vi "Example_OE2052 Control.vi"() -> ()   [LabVIEW 2011]
uses:
  <vilib>/Utility/error.llb/DialogType.ctl
panel:
  out "B_Freq":dbl
  out "B_θ":dbl
  out "B_R":dbl
  out "B_Overload":bool
  in  "Sample count":u32
  out "Zero Data?":bool
  in  "buffer":u8
  out "Queue out":errorcluster caption="error out"
  out "Queue output":refnum<queue>
  in  "IP Address":string
  in  "Timeout":u32=100
  in  "Port":u32=10001
  out "B_PLL Lock":bool
  in  "Remote Mode":u16(ring) items=["USB"=0, "RS232"=1, "Ethernet"=3]
  out "A_Freq":dbl
  out "A_θ":dbl
  out "A_R":dbl
  out "A_PLL Lock":bool
  out "A_Overload":bool
  out "Error":string
  out "Serial Versions":string
  in  "Table":T1(tab) caption="选项卡控件"
  in  "OE2052_Configure Input Filter":T2={"Input Source"=0, "Input Impedance"=0, "Input Coupling "=0, "Sample Mode"=0, "Channel"=1, "Input Range"=0} {"Input Range" items=["1.3V", "200mV", "50mV", "10mV", "2mV", "500uV", "100uV"]; "Channel" items=["A"=1, "B"=2]; "Sample Mode" items=["HF", "LF"]; "Input Coupling" items=["AC", "DC"]; "Input Impedance" items=["50Ω", "10MΩ"]; "Input Source" items=["A", "A-B"]}
  in  "OE2052_Configure Ref Phase":T3={"Reference Source"=0, "Internal Frequency(Hz)"=1000.0, "Reference Phase"=0.0, "Reference Slope"=0, "Channel"=1, "Reference Range"=0} {"Reference Range" items=["HIGH", "LOW"]; "Channel" items=["A"=1, "B"=2]; "Reference Slope" items=["SINEDC", "SINE", "TTL"]; "Reference Phase" min=-180.0 max=180.0 format="%#.2g"; "Internal Frequency(Hz)" min=1e-05 max=60000000.0 format="%#.3f"; "Reference Source" items=["External", "Internal", "Self"]}
  in  "OE2052_Configure \nGain TC":T4={"Time Constant "=20.0, "Low Pass Filter Slope "=3, "Enable Sync Filter "=0, "Channel"=1} {"Channel" items=["A"=1, "B"=2]; "Enable Sync Filter" items=["OFF", "ON"]; "Low Pass Filter Slope" items=["6 dB/oct", "12 dB/oct", "18 db/oct", "24 dB/oct", "30 dB/oct", "36 dB/oct", "42 dB/oct", "48 dB/oct"]; "Time Constant" min=1e-07 max=100.0 format="%#.3f"}
  in  "OE2052_Configure Channel Out":T5={"Channel Output"=0, "Channel Source"=0, "Offset(%)"=0.0, "Expand"=1, "AUX OUT"=1.0, "Sensitivity "=24} {"Sensitivity" items=["1 nV/fA", "2 nV/fA", "5 nV/fA", "10 nV/fA", "20 nV/fA", "50 nV/fA", "100 nV/fA", "200 nV/fA", "500 nV/fA", "1 uV/pA", "2 uV/pA", "5 uV/pA", "10 uV/pA", "20 uV/pA", "50 uV/pA", "100 uV/pA", "200 uV/pA", "500 uV/pA", "1 mV/nA", "2 mV/nA", "5 mV/nA", "10 mV/nA", "20 mV/nA", "50 mV/nA", "100 mV/nA", "200 mV/nA", "500 mV/nA", "1 V/uA"]; "AUX OUT" min=-10.0 max=10.0 format="%#.3g"; "Expand" min=1 max=10000; "Offset(%)" min=-100.0 max=100.0 format="%#_5g"; "Channel Source" items=["AUXOUT", "X1", "Y1", "R1", "θ1", "X2", "Y2", "R2", "θ2", "Frequency1", "Frequency2", "AUX-IN1", "AUX-IN2", "AUX-IN3", "AUX-IN4"]; "Channel Output" items=["CH1", "CH2", "CH3", "CH4"]}
  in  "OE2052_Configure Sine Out":T6={"SineOut Amplitude (V)"=1.0, "SineOut Offset(V) "=1.0, "SineOut Unit"=0, "SineOut Impedance"=0, "Channel"=1, "SineOut Mode"=0} {"SineOut Mode" items=["OFF", "Fixed"]; "Channel" items=["A"=1, "B"=2]; "SineOut Impedance" items=["50Ω", "HiZ"]; "SineOut Unit" items=["VPP", "VRMS"]; "SineOut Offset(V)" min=-2.5 max=2.5 format="%#.3g"; "SineOut Amplitude (V)" min=1e-06 max=1.5 format="%#.3g"}
  in  "OE2052_Configure Demodulator":T7={"Mode"=0, "Harmonic"=1, "Channel"=1} {"Channel" items=["A"=1, "B"=2]; "Harmonic" min=1; "Mode" items=["Harmonic"]}
  in  "OE2052_Auto Setting":T8={"Auto Range"=FALSE, "Auto Offest"=FALSE, "Auto Phase"=FALSE, "channel"=1} {"channel" items=["A"=1, "B"=2]}
  in  "Save Button":bool
  in  "file path":path
  in  "Sample Rate(S)":dbl=0.1 min=0.001 max=100.0
  out "Status":string
  in  "Connect":bool
  in  "VISA resource name":refnum<visa-resource-name>
  in  "Baud Rate (115200)":u32=921600
  # "Tel          :   +86-020-84133345\nWebsite  :   www.ssi-instrument.com\nE-mail     :   support@si-instrument.com"
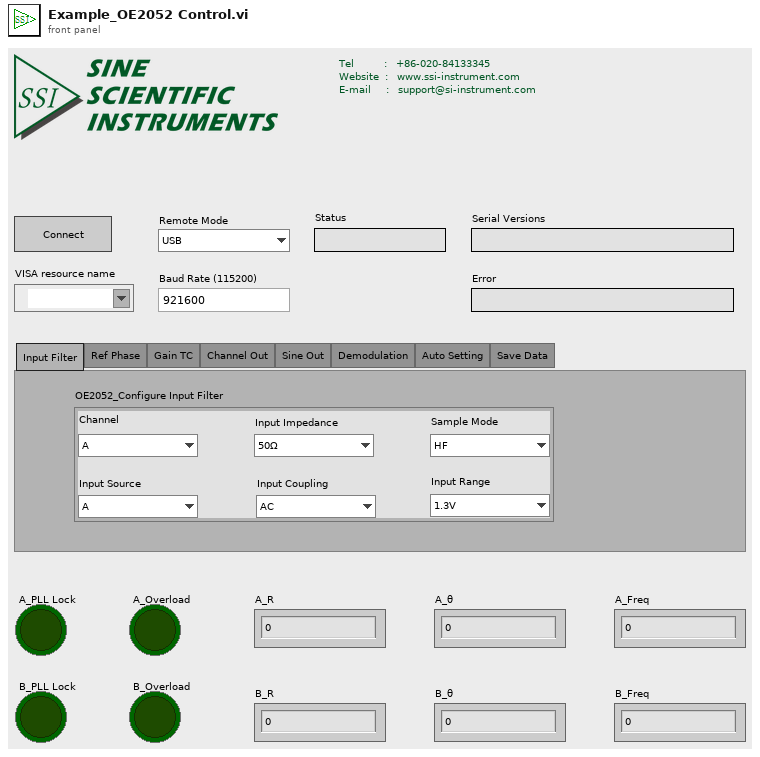
[diagram p1: front panel]
types:
  T1 = enum32{"Input Filter", "Ref Phase", "Gain TC", "Channel Out", "Sine Out", "Demodulation", "Auto Setting", "Save Data"}
  T2 = cluster{"Input Source":u16, "Input Impedance":u16, "Input Coupling ":u16, "Sample Mode":u16, "Channel":u16, "Input Range":u16}
  T3 = cluster{"Reference Source":u16, "Internal Frequency(Hz)":dbl, "Reference Phase":dbl, "Reference Slope":u16, "Channel":u16, "Reference Range":u16}
  T4 = cluster{"Time Constant ":dbl, "Low Pass Filter Slope ":u8, "Enable Sync Filter ":u16, "Channel":u16}
  T5 = cluster{"Channel Output":u16, "Channel Source":u16, "Offset(%)":dbl, "Expand":u16, "AUX OUT":dbl, "Sensitivity ":u16}
  T6 = cluster{"SineOut Amplitude (V)":dbl, "SineOut Offset(V) ":dbl, "SineOut Unit":u8, "SineOut Impedance":u8, "Channel":u16, "SineOut Mode":u8}
  T7 = cluster{"Mode":u16, "Harmonic":u16, "Channel":u16}
  T8 = cluster{"Auto Range":bool, "Auto Offest":bool, "Auto Phase":bool, "channel":u16}
  T9 = enum16{"OE1022", "OE1022D", "OE1201", "OE2031&OE2041", "OE1311&OE1351", "OE2052"}
  T10 = cluster{"Port":u32, "Timeout":u32, "IP Address":string}
  T11 = cluster{"A_PLL Lock":bool, "A_Overload":bool, "B_PLL Lock":bool, "B_Overload":bool}
  T12 = cluster{"A_X":dbl, "A_Y":dbl, "A_R":dbl, "A_θ":dbl, "A_Freq":dbl, "B_X":dbl, "B_Y":dbl, "B_R":dbl, "B_θ":dbl, "B_Freq":dbl, "Aux_In1":dbl, "Aux_In2":dbl, "Aux_In3":dbl, "Aux_In4":dbl}
  T13 = typedef "DialogType.ctl" = u16
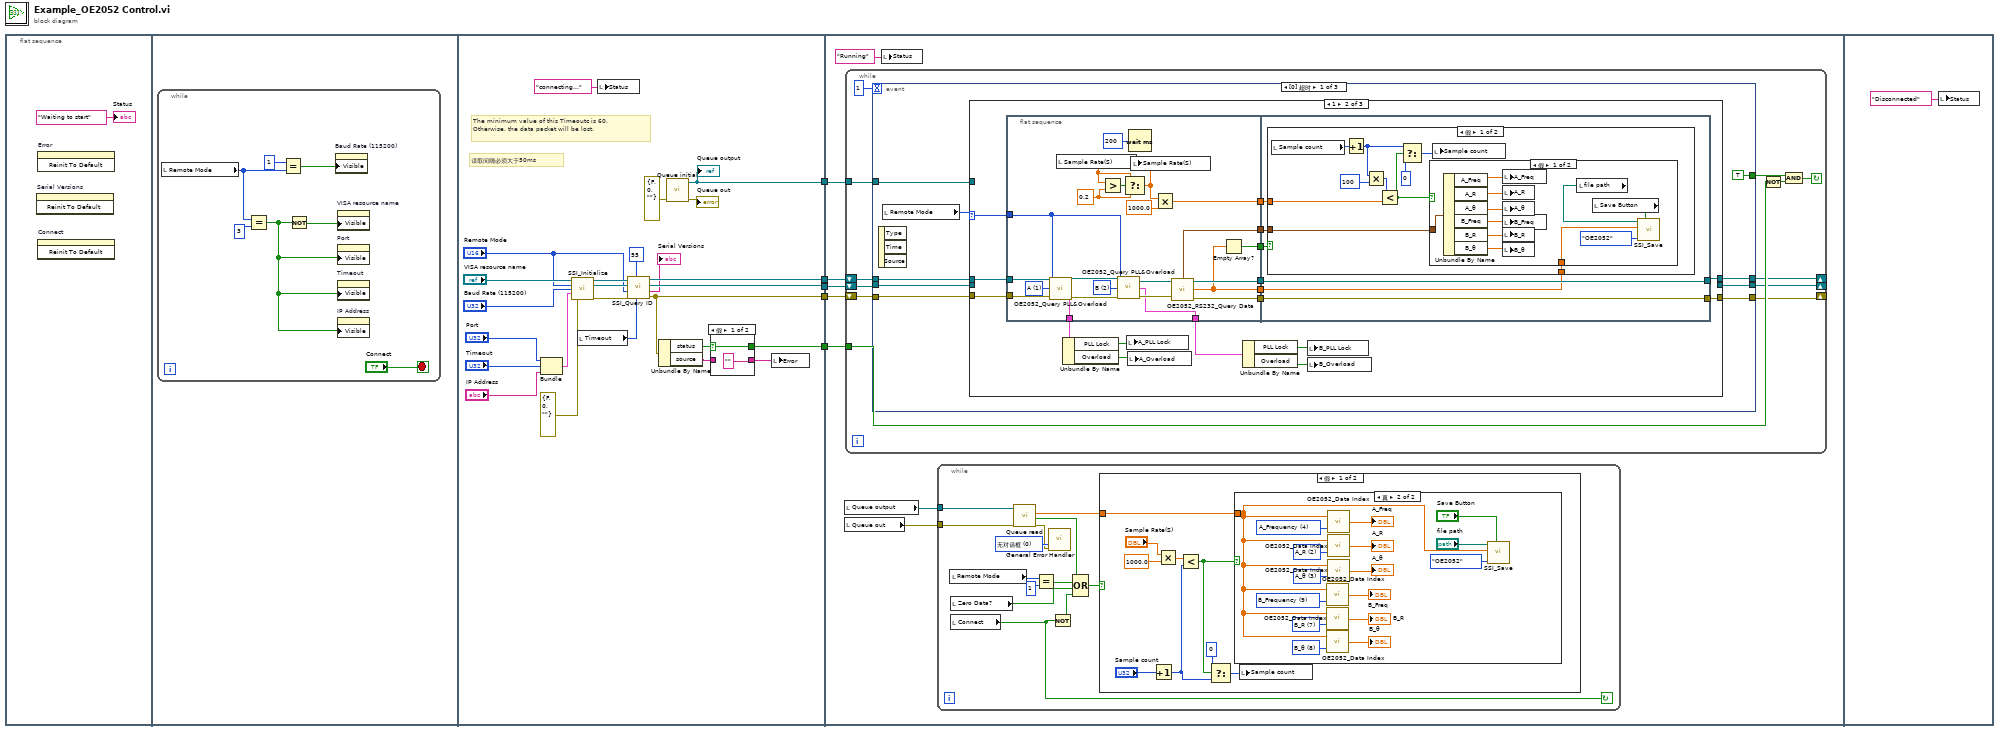
[diagram p0: block diagram]
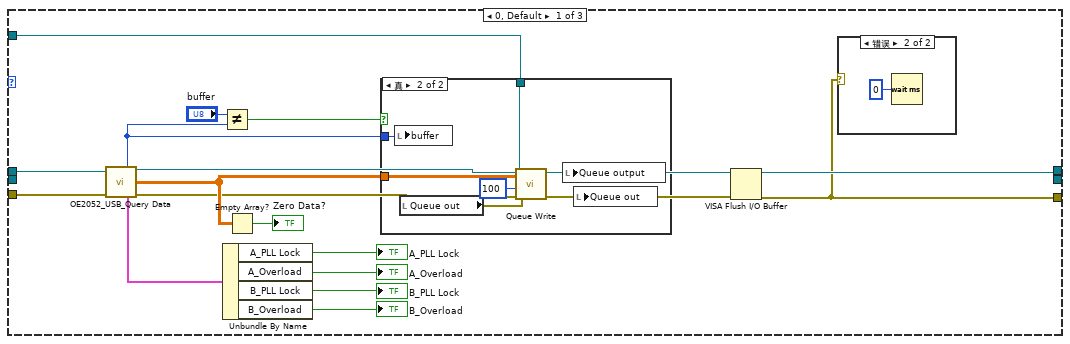
[diagram p5: hidden frame]
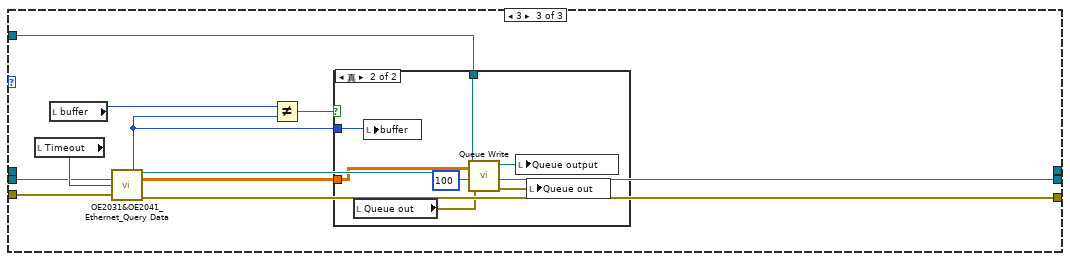
[diagram p10: hidden frame]
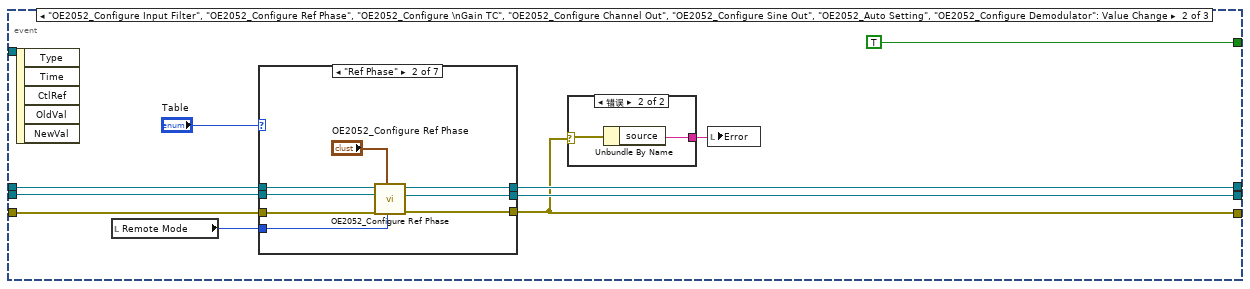
[diagram p12: hidden frame]
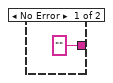
[diagram p13: hidden frame]
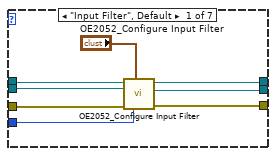
[diagram p14: hidden frame]
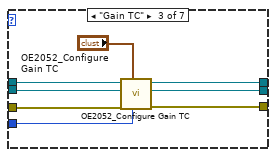
[diagram p15: hidden frame]
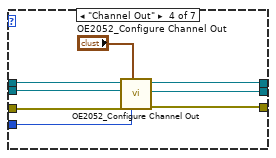
[diagram p16: hidden frame]
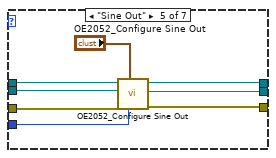
[diagram p17: hidden frame]
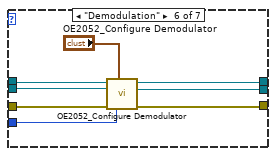
[diagram p18: hidden frame]
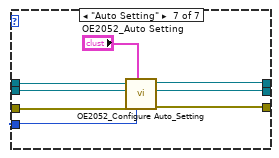
[diagram p19: hidden frame]
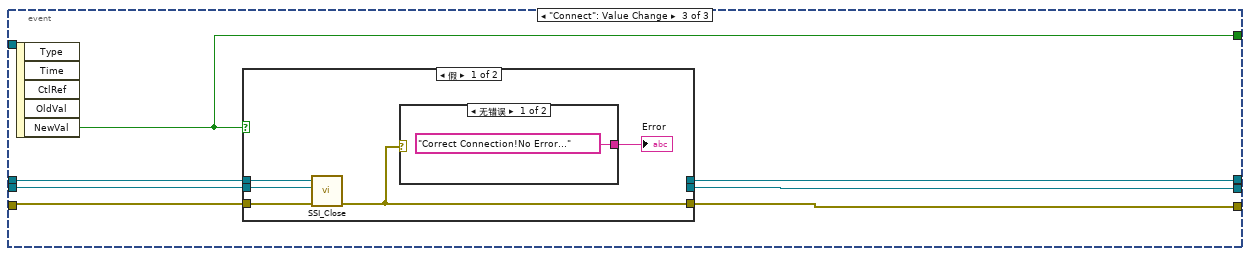
[diagram p20: hidden frame]
diagram:
  n1 = flat-sequence {
    tunnel: [w32] -> w5
    tunnel: [w31] -> w4
    tunnel: [w28] -> w3
    tunnel: [w25] -> w2
    tunnel: [w16] -> w1
    tunnel: w5 -> [w49]
    tunnel: w4 -> [w48]
    tunnel: w3 -> [w47]
    tunnel: w2 -> [w46]
    tunnel: w1 -> [w43]
    frame #0 {
      n2 = invoke on="Serial Versions" class="Str" method="Reinit To Default"() -> ()  [unwired: 3 in, 3 out]
      n3 = invoke on="Error" class="Str" method="Reinit To Default"() -> ()  [unwired: 3 in, 3 out]
      n4 = invoke on="Connect" class="Bool (严格)" method="Reinit To Default"() -> ()  [unwired: 3 in, 3 out]
      "Status" <- "Waiting to start" ("status")
    }
    frame #1 {
      n5 = while {
        stop <- "Connect" stop-if-true
        n6 = local read "Remote Mode"() -> (w8:u16)
        n7 = Equal?(x=w8, y=u16 3) -> (x = y?=w10:bool)
        n8 = Equal?(x=u16 1, y=w8) -> (x = y?=w7:bool)
        n9 = Not(x=w10) -> (.not. x?=w11:bool)
        n10 = property on="Baud Rate (115200)" class="DigNum (严格)"("Visible"=w7) -> ()  [unwired: 2 in, 2 out]
        n11 = property on="VISA resource name" class="VISAName"("Visible"=w11) -> ()  [unwired: 2 in, 2 out]
        n12 = property on="Port" class="DigNum (严格)"("Visible"=w10) -> ()  [unwired: 2 in, 2 out]
        n13 = property on="Timeout" class="DigNum (严格)"("Visible"=w10) -> ()  [unwired: 2 in, 2 out]
        n14 = property on="IP Address" class="Str"("Visible"=w10) -> ()  [unwired: 2 in, 2 out]
      }
    }
    frame #2 {
      # "读取间隔必须大于50ms"
      # "The minimum value of this Timeoutc is 60. \nOtherwise, the data packet will be lost."
      n15 = Bundle("Port"="Port", "Timeout"="Timeout", "IP Address"="IP Address") -> (w20:T10)  [unwired: 1 in]
      n16 = call "SSI_Initialize.vi"("VISA resource name"="VISA resource name", "Remote Mode"="Remote Mode", "baud rate (921600)"="Baud Rate (115200)", "Ethernet"=w20, "error in (no error)"=errorcluster {"status"=FALSE, "code"=0, "source"=""}) -> ("VISA resource name out"=w36:refnum<visa-resource-name>, "connection ID(Ethernet)"=w35:refnum<k5>, "error out"=w34:errorcluster)  [unwired: 8 in]
      n17 = local read "Timeout"() -> (w19:u32)
      n18 = local write "Status"("connecting..." ("status")) -> ()
      n19 = call "SSI_Query ID.vi"("Timeout"=w19, "Number of bytes"=u32 55, "Error in (no error)"=w34, "Remote Mode"="Remote Mode", "Connection ID in"=w35, "VISA resource name"=w36) -> ("Error out"=w28:errorcluster, "Read Buffer"=→"Serial Versions":string, "Connection ID out"=w31:refnum<k5>, "VISA resource  out"=w32:refnum<visa-resource-name>)  [unwired: 2 in]
      n20 = Unbundle By Name(w28) -> ("status"=w27:bool, "source"=w26:string)
      n21 = call "Queue initial.vi"("Error in (no error)"=errorcluster {"status"=FALSE, "code"=0, "source"=""}) -> ("Error out"=→"Queue out":errorcluster, "Queue output"=w16:refnum<queue>)  [unwired: 9 in]
      "Queue output" <- w16
      n22 = case shown="假" w27 {
        selector: w27 -> [w40 w42]
        tunnel: [w40 w42] -> w25
        tunnel: ["" w41] -> w24
        tunnel: w26 -> [_ w41]
        frame False {
        }
        frame True {
        }
      }
      n23 = local write "Error"(w24) -> ()
    }
    frame #3 {
      n24 = local read "Queue output"() -> (w45:refnum<queue>)
      n25 = local read "Queue out"() -> (w44:errorcluster)
      n26 = while {
        tunnel: w46 -> [w96]
        tunnel: w43 -> [w92]
        shift-right: [w89] -> _
        shift-left: w47 -> [w93]
        shift-right: [w90] -> _
        shift-left: w48 -> [w94]
        shift-right: [w91] -> _
        shift-left: w49 -> [w95]
        stop <- w97 continue-if-true
        n27 = event shown="[0] 超时" {
          selector: _ -> [_ _ _]
          dyn-events: _ -> [_ _ _]
          timeout: 1 -> [_ _ _]
          tunnel: [TRUE ("Stop") TRUE ("Stop") w288] -> w98
          tunnel: [w109 w219 w291] -> w89
          tunnel: [w108 w224 w290] -> w91
          tunnel: [w107 w223 w289] -> w90
          tunnel: w95 -> [w103 w227 w294]
          tunnel: w94 -> [w101 w226 w293]
          tunnel: w93 -> [w102 w225 w292]
          tunnel: w92 -> [w104 _ _]
          event Timeout {
            n28 = event-data() -> ()  [unwired: 1 in, 3 out]
            n29 = local read "Remote Mode"() -> (w105:u16)
            n30 = case shown="1" w105 {
              selector: w105 -> [_ w147 _]
              tunnel: [w115 w149 w209] -> w109
              tunnel: [w118 w148 _] -> w108
              tunnel: [_ _ w210] -> w107
              tunnel: w104 -> [w126 _ w208]
              tunnel: w103 -> [w117 w151 _]
              tunnel: w102 -> [w116 w150 w202]
              tunnel: w101 -> [_ _ w203]
              frame 0, Default {
                n31 = call "OE2052_USB_Query Data.vi"("VISA resource name"=w117, "Error in (no error)"=w116) -> ("Buffer Count"=w123:u8, "VISA resource  out"=w120:refnum<visa-resource-name>, "Total Data Array"=w122:dbl[][], "A&B_PLL&Overload"=w110:T11, "Error out"=w119:errorcluster)  [unwired: 7 in, 2 out]
                n32 = Not Equal?(x="buffer", y=w123) -> (x != y?=w124:bool)
                n33 = Unbundle By Name(w110) -> ("A_PLL Lock"=→"A_PLL Lock":bool, "A_Overload"=→"A_Overload":bool, "B_PLL Lock"=→"B_PLL Lock":bool, "B_Overload"=→"B_Overload":bool)
                n34 = Empty Array?(array=w122) -> (empty?=→"Zero Data?":bool)
                n35 = case shown="真" w124 {
                  tunnel: w122 -> [_ w128]
                  tunnel: w126 -> [_ w133]
                  tunnel: w123 -> [_ w129]
                  frame False {
                  }
                  frame True {
                    n36 = local write "buffer"(w129) -> ()
                    n37 = local read "Queue out"() -> (w130:errorcluster)
                    n38 = call "Queue Write.vi"("Error in (no error)"=w130, "Group Count"=100, "Input Array"=w128, "Queue Input"=w133) -> ("Error out"=w131:errorcluster, "Queue output"=w132:refnum<queue>)  [unwired: 6 in]
                    n39 = local write "Queue output"(w132) -> ()
                    n40 = local write "Queue out"(w131) -> ()
                  }
                }
                n41 = VISA Flush I/O Buffer(VISA resource name=w120, error in (no error)=w119) -> (VISA resource name out=w118:refnum<visa-resource-name>, error out=w115:errorcluster)  [unwired: 1 in]
                n42 = case shown="错误" w115 {
                  frame No Error {
                  }
                  frame Error {
                    n43 = Wait (ms)(milliseconds to wait=u32 0 ("等待时间（毫秒）")) -> ()  [unwired: 1 out]
                  }
                }
              }
              frame 1 {
                n44 = flat-sequence {
                  tunnel: [w166] -> w146
                  tunnel: [w167] -> w145
                  tunnel: [w170] -> w144
                  tunnel: [w169] -> w143
                  tunnel: [w165] -> w142
                  tunnel: [w161] -> w141
                  tunnel: w151 -> [w160]
                  tunnel: w150 -> [w159]
                  tunnel: w147 -> [w154]
                  tunnel: [w153] -> w140
                  tunnel: [w152] -> w137
                  tunnel: w146 -> [w179]
                  tunnel: w145 -> [w180]
                  tunnel: [w180] -> w148
                  tunnel: [w179] -> w149
                  tunnel: w144 -> [w176]
                  tunnel: w143 -> [w175]
                  tunnel: w142 -> [w177]
                  tunnel: w141 -> [w178]
                  frame #0 {
                    w155 = u16 2 items=["A"=1, "B"=2] ("channel")
                    w156 = u16 1 items=["A"=1, "B"=2] ("channel")
                    w173 = 0.2 ("y")
                    n45 = call "OE2052_Query PLL&Overload.vi"("VISA resource name"=w160, "channel"=w156, "Remote Mode"=w154, "Error in (no error)"=w159) -> ("VISA resource  out"=w157:refnum<visa-resource-name>, "OE2052_Query \nPLL&Overload"=w153:cluster{"PLL Lock":bool, "Overload":bool}, "Error out"=w158:errorcluster)  [unwired: 7 in, 2 out]
                    n46 = local read "Sample Rate(S)"() -> (w168:dbl)
                    n47 = Greater?(x=w168, y=w173) -> (0:w172:bool)
                    n48 = call "OE2052_Query PLL&Overload.vi"("VISA resource name"=w157, "channel"=w155, "Remote Mode"=w154, "Error in (no error)"=w158) -> ("VISA resource  out"=w164:refnum<visa-resource-name>, "OE2052_Query \nPLL&Overload"=w152:cluster{"PLL Lock":bool, "Overload":bool}, "Error out"=w163:errorcluster)  [unwired: 7 in, 2 out]
                    n49 = Select(t=w168, s=w172, f=w173) -> (s? t:f=w171:dbl)
                    n50 = Wait (ms)(milliseconds to wait=u32 200 ("等待时间（毫秒）")) -> ()  [unwired: 1 out]
                    n51 = local write "Sample Rate(S)"(w171) -> ()
                    n52 = Multiply(x=w171, y=1000.0) -> (x*y=w169:dbl)
                    n53 = call "OE2052_RS232_Query Data.vi"("VISA resource name"=w164, "Error in (no error)"=w163) -> ("VISA resource  out"=w167:refnum<visa-resource-name>, "Data Array"=w161:dbl[], "Parameter Values"=w165:T12, "Error out"=w166:errorcluster)  [unwired: 9 in, 1 out]
                    n54 = Empty Array?(array=w161) -> (empty?=w170:bool)
                  }
                  frame #1 {
                    n55 = case shown="假" w176 {
                      tunnel: w178 -> [w190 _]
                      tunnel: w177 -> [w189 _]
                      tunnel: w175 -> [w185 _]
                      frame False {
                        n56 = local read "Sample count"() -> (w188:u32)
                        n57 = Increment(x=w188) -> (x+1=w184:u32)
                        n58 = Multiply(x=w184, y=u32 100) -> (x*y=w186:u32)
                        n59 = Less?(x=w186, y=w185) -> (x < y?=w183:bool)
                        n60 = Select(t=w184, s=w183, f=0) -> (s? t:f=w182:u32)
                        n61 = case shown="假" w183 {
                          tunnel: w189 -> [w201 _]
                          tunnel: w190 -> [w197 _]
                          frame False {
                            n62 = Unbundle By Name(w201) -> ("A_Freq"=w200:dbl, "A_R"=w199:dbl, "A_θ"=w198:dbl, "B_Freq"=w193:dbl, "B_R"=w191:dbl, "B_θ"=w192:dbl)
                            n63 = local write "A_Freq"(w200) -> ()
                            n64 = local write "A_R"(w199) -> ()
                            n65 = local write "A_θ"(w198) -> ()
                            n66 = local write "B_Freq"(w193) -> ()
                            n67 = local write "B_R"(w191) -> ()
                            n68 = local write "B_θ"(w192) -> ()
                            n69 = local read "file path"() -> (w196:path)
                            n70 = local read "Save Button"() -> (w195:bool)
                            n71 = call "SSI_Save.vi"("file path (dialog if empty)"=w196, "1D data"=w197, "Instrument Mode"=T9."OE2052", "Save Button"=w195) -> ()  [unwired: 7 in]
                          }
                          frame True {
                          }
                        }
                        n72 = local write "Sample count"(w182) -> ()
                      }
                      frame True {
                      }
                    }
                  }
                }
                n73 = Unbundle By Name(w140) -> ("PLL Lock"=w138:bool, "Overload"=w139:bool)
                n74 = local write "A_PLL Lock"(w138) -> ()
                n75 = local write "A_Overload"(w139) -> ()
                n76 = Unbundle By Name(w137) -> ("PLL Lock"=w136:bool, "Overload"=w135:bool)
                n77 = local write "B_PLL Lock"(w136) -> ()
                n78 = local write "B_Overload"(w135) -> ()
              }
              frame 3 {
                n79 = local read "Timeout"() -> (w211:u32)
                n80 = local read "buffer"() -> (w206:u8)
                n81 = call "OE2031&OE2041_Ethernet_Query Data.vi"("Connection ID in"=w203, "Timeout"=w211, "Error in (no error)"=w202) -> ("Buffer Count"=w205:u8, "Connection ID out"=w210:refnum<k5>, "Total Data Array"=w204:dbl[][], "Error out"=w209:errorcluster)  [unwired: 5 in, 4 out]
                n82 = Not Equal?(x=w206, y=w205) -> (x != y?=w207:bool)
                n83 = case shown="真" w207 {
                  tunnel: w208 -> [_ w217]
                  tunnel: w205 -> [_ w213]
                  tunnel: w204 -> [_ w212]
                  frame False {
                  }
                  frame True {
                    n84 = local read "Queue out"() -> (w214:errorcluster)
                    n85 = local write "buffer"(w213) -> ()
                    n86 = call "Queue Write.vi"("Error in (no error)"=w214, "Group Count"=100, "Input Array"=w212, "Queue Input"=w217) -> ("Error out"=w215:errorcluster, "Queue output"=w216:refnum<queue>)  [unwired: 6 in]
                    n87 = local write "Queue output"(w216) -> ()
                    n88 = local write "Queue out"(w215) -> ()
                  }
                }
              }
            }
          }
          event "OE2052_Configure Input Filter", "OE2052_Configure Ref Phase", "OE2052_Configure \nGain TC", "OE2052_Configure Channel Out", "OE2052_Configure Sine Out", "OE2052_Auto Setting", "OE2052_Configure Demodulator": Value Change {
            n89 = event-data() -> ()  [unwired: 1 in, 5 out]
            n90 = local read "Remote Mode"() -> (w222:u16)
            n91 = case shown="\"Ref Phase\"" "Table" {
              tunnel: w227 -> [w238 w247 w255 w260 w267 w276 w287]
              tunnel: w226 -> [w237 w246 w253 w261 w266 w277 w286]
              tunnel: w225 -> [w239 w245 w254 w263 w271 w279 w285]
              tunnel: [w234 w244 w251 w257 w268 w275 w283] -> w224
              tunnel: [w235 w243 w252 w259 w270 w274 w281] -> w219
              tunnel: [w236 w242 w250 w258 w269 w273 w282] -> w223
              tunnel: w222 -> [w233 w241 w249 w262 w265 w278 w284]
              frame "Input Filter", Default {
                n92 = call "OE2052_Configure Input Filter.vi"("OE2052_Configure Input Filter"="OE2052_Configure Input Filter", "Error in (no error)"=w239, "Remote Mode"=w233, "Connection ID in"=w237, "VISA resource name"=w238) -> ("Error out"=w235:errorcluster, "Connection ID out"=w236:refnum<k5>, "VISA resource  out"=w234:refnum<visa-resource-name>)  [unwired: 3 in, 1 out]
              }
              frame "Ref Phase" {
                n93 = call "OE2052_Configure Ref Phase.vi"("OE2052_Configure Ref Phase"="OE2052_Configure Ref Phase", "Error in (no error)"=w245, "Remote Mode"=w241, "Connection ID in"=w246, "VISA resource name"=w247) -> ("Error out"=w243:errorcluster, "Connection ID out"=w242:refnum<k5>, "VISA resource  out"=w244:refnum<visa-resource-name>)  [unwired: 3 in, 1 out]
              }
              frame "Gain TC" {
                n94 = call "OE2052_Configure Gain TC.vi"("OE2052_Configure \nGain TC"="OE2052_Configure \nGain TC", "Error in (no error)"=w254, "Remote Mode"=w249, "Connection ID in"=w253, "VISA resource name"=w255) -> ("Error out"=w252:errorcluster, "Connection ID out"=w250:refnum<k5>, "VISA resource  out"=w251:refnum<visa-resource-name>)  [unwired: 3 in, 1 out]
              }
              frame "Channel Out" {
                n95 = call "OE2052_Configure Channel Out.vi"("OE2052_Configure Channel Out"="OE2052_Configure Channel Out", "Error in (no error)"=w263, "Remote Mode"=w262, "Connection ID in"=w261, "VISA resource name"=w260) -> ("Error out"=w259:errorcluster, "Connection ID out"=w258:refnum<k5>, "VISA resource  out"=w257:refnum<visa-resource-name>)  [unwired: 3 in, 1 out]
              }
              frame "Sine Out" {
                n96 = call "OE2052_Configure Sine Out.vi"("OE2052_Configure Sine Out"="OE2052_Configure Sine Out", "Error in (no error)"=w271, "Remote Mode"=w265, "Connection ID in"=w266, "VISA resource name"=w267) -> ("Error out"=w270:errorcluster, "Connection ID out"=w269:refnum<k5>, "VISA resource  out"=w268:refnum<visa-resource-name>)  [unwired: 3 in, 1 out]
              }
              frame "Demodulation" {
                n97 = call "OE2052_Configure Demodulator.vi"("OE2052_Configure Demodulator"="OE2052_Configure Demodulator", "Error in (no error)"=w279, "Remote Mode"=w278, "Connection ID in"=w277, "VISA resource name"=w276) -> ("Error out"=w274:errorcluster, "Connection ID out"=w273:refnum<k5>, "VISA resource  out"=w275:refnum<visa-resource-name>)  [unwired: 3 in, 1 out]
              }
              frame "Auto Setting" {
                n98 = call "OE2052_Configure Auto_Setting.vi"("OE2052_Auto Setting"="OE2052_Auto Setting", "Error in (no error)"=w285, "Remote Mode"=w284, "Connection ID in"=w286, "VISA resource name"=w287) -> ("Error out"=w281:errorcluster, "Connection ID out"=w282:refnum<k5>, "VISA resource  out"=w283:refnum<visa-resource-name>)  [unwired: 3 in, 1 out]
              }
            }
            n99 = case shown="错误" w219 {
              selector: w219 -> [_ w231]
              tunnel: ["" ("source") w230] -> w220
              frame No Error {
              }
              frame Error {
                n100 = Unbundle By Name(w231) -> ("source"=w230:string)
              }
            }
            n101 = local write "Error"(w220) -> ()
          }
          event "Connect": Value Change {
            n102 = event-data() -> ("NewVal"=w288:bool)  [unwired: 1 in, 4 out]
            n103 = case shown="假" w288 {
              tunnel: w294 -> [w299 w304]
              tunnel: w293 -> [w298 w303]
              tunnel: w292 -> [w297 w305]
              tunnel: [w296 w305] -> w291
              tunnel: [_ w304] -> w290
              tunnel: [_ w303] -> w289
              frame False {
                n104 = call "SSI_Close.vi"("Error in (no error)"=w297, "Connection ID in"=w298, "VISA resource name"=w299) -> ("Error out"=w296:errorcluster)  [unwired: 4 in]
                n105 = case shown="无错误" w296 {
                  selector: w296 -> [_ w302]
                  tunnel: ["Correct Connection!No Error..." ("source") w301] -> w295
                  frame No Error {
                  }
                  frame Error {
                    n106 = Unbundle By Name(w302) -> ("source"=w301:string)
                  }
                }
                "Error" <- w295
              }
              frame True {
              }
            }
          }
        }
        n107 = Not(x=w96) -> (.not. x?=w99:bool)
        n108 = And(x=w98, y=w99) -> (x .and. y?=w97:bool)
      }
      n109 = local write "Status"("Running" ("status")) -> ()
      n110 = while {
        tunnel: w45 -> [w56]
        tunnel: w44 -> [w55]
        stop <- w51 continue-if-true
        w58 = T13 0 items=["无对话框", "确定信息", "继续或停止信息", "确定信息＋警告", "继续/停止+警告"] ("type of dialog (OK msg:1)")
        n111 = local read "Remote Mode"() -> (w63:u16)
        n112 = local read "Zero Data?"() -> (w59:bool)
        n113 = local read "Connect"() -> (w51:bool)
        n114 = call "Queue read.vi"("Error in (no error)"=w55, "Queue Input"=w56) -> ("Error out"=w57:errorcluster, "Timeout？"=w53:bool, "Output Array"=w54:sgl[])  [unwired: 7 in]
        n115 = Equal?(x=w63, y=u16 1) -> (x = y?=w60:bool)
        n116 = call <vilib>:"General Error Handler.vi"("type of dialog (OK msg:1)"=w58, "error in (no error)"=w57) -> ()  [unwired: 9 in, 5 out]
        n117 = Not(x=w51) -> (.not. x?=w52:bool)
        n118 = Compound Arithmetic op=OR(w53, w60, w59, w52) -> (w61:bool)
        n119 = case shown="假" w61 {
          tunnel: w54 -> [w72 _]
          frame False {
            n120 = Increment(x="Sample count") -> (x+1=w66:u32)
            n121 = Multiply(x="Sample Rate(S)", y=1000.0) -> (x*y=w70:dbl)
            n122 = Less?(x=w70, y=w66) -> (x < y?=w67:bool)
            n123 = Select(t=0, s=w67, f=w66) -> (s? t:f=w65:u32)
            n124 = case shown="真" w67 {
              tunnel: w72 -> [_ w76]
              frame False {
              }
              frame True {
                w77 = u16 8 items=["A_X", "A_Y", "A_R", "A_θ", "A_Frequency", "B_X", "B_Y", "B_R", "B_θ", "B_Frequency"] ("Parameter Type")
                w78 = u16 7 items=["A_X", "A_Y", "A_R", "A_θ", "A_Frequency", "B_X", "B_Y", "B_R", "B_θ", "B_Frequency"] ("Parameter Type")
                w79 = u16 9 items=["A_X", "A_Y", "A_R", "A_θ", "A_Frequency", "B_X", "B_Y", "B_R", "B_θ", "B_Frequency"] ("Parameter Type")
                w80 = u16 3 items=["A_X", "A_Y", "A_R", "A_θ", "A_Frequency", "B_X", "B_Y", "B_R", "B_θ", "B_Frequency"] ("Parameter Type")
                w81 = u16 2 items=["A_X", "A_Y", "A_R", "A_θ", "A_Frequency", "B_X", "B_Y", "B_R", "B_θ", "B_Frequency"] ("Parameter Type")
                w82 = u16 4 items=["A_X", "A_Y", "A_R", "A_θ", "A_Frequency", "B_X", "B_Y", "B_R", "B_θ", "B_Frequency"] ("Parameter Type")
                n125 = call "OE2052_Data Index.vi"("Parameter Type"=w79, "Input Date Array"=w76) -> ("Parameter"=→"B_Freq":dbl)
                n126 = call "OE2052_Data Index.vi"("Parameter Type"=w78, "Input Date Array"=w76) -> ("Parameter"=→"B_R":dbl)
                n127 = call "OE2052_Data Index.vi"("Parameter Type"=w77, "Input Date Array"=w76) -> ("Parameter"=→"B_θ":dbl)
                n128 = call "OE2052_Data Index.vi"("Parameter Type"=w82, "Input Date Array"=w76) -> ("Parameter"=→"A_Freq":dbl)
                n129 = call "OE2052_Data Index.vi"("Parameter Type"=w81, "Input Date Array"=w76) -> ("Parameter"=→"A_R":dbl)
                n130 = call "OE2052_Data Index.vi"("Parameter Type"=w80, "Input Date Array"=w76) -> ("Parameter"=→"A_θ":dbl)
                n131 = call "SSI_Save.vi"("file path (dialog if empty)"="file path", "1D data"=w76, "Instrument Mode"=T9."OE2052", "Save Button"="Save Button") -> ()  [unwired: 7 in]
              }
            }
            n132 = local write "Sample count"(w65) -> ()
          }
          frame True {
          }
        }
      }
    }
    frame #4 {
      n133 = local write "Status"("Disconnected" ("status")) -> ()
    }
  }
